vi "SamePrototype.vi"(4 "String To Append":string, 5 "Number To Multiply":dbl format="%.2f", 6 "Cluster In":T1 {"Numeric" format="%.2f"}, 7 "Array In":dbl[](array[numeric]) format="%.2f", 8 "String In":string, 9 "Numeric In":dbl format="%.2f") -> (0 "Cluster Out":T1 {"Numeric" format="%.2f"}, 1 "Array Out":dbl[](array[numeric]) format="%.2f", 2 "String Out":string, 3 "Numeric Out":dbl format="%.2f")   [LabVIEW 2012]
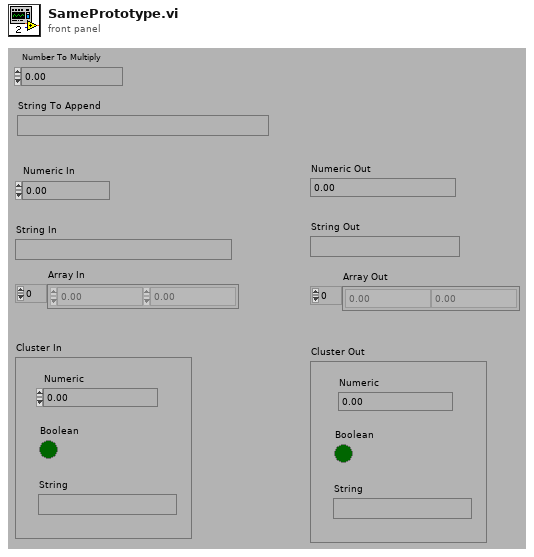
[diagram p1: front panel]
types:
  T1 = cluster{"Numeric":dbl, "Boolean":bool, "String":string}
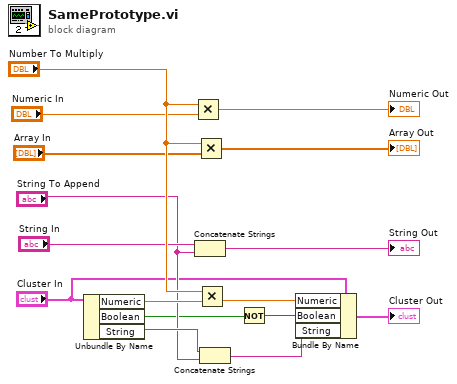
[diagram p0: block diagram]
diagram:
  n1 = Unbundle By Name("Cluster In") -> ("Numeric"=w15:dbl, "Boolean"=w7:bool, "String"=w9:string)
  n2 = Multiply(x="Number To Multiply", y="Numeric In") -> (x*y=→"Numeric Out":dbl)
  n3 = Concatenate Strings("String In", "String To Append") -> (→"String Out":string)
  n4 = Multiply(x="Number To Multiply", y="Array In") -> (x*y=→"Array Out":dbl[])
  n5 = Multiply(x="Number To Multiply", y=w15) -> (x*y=w4:dbl)
  n6 = Concatenate Strings(w9, "String To Append") -> (w3:string)
  n7 = Not(x=w7) -> (.not. x?=w5:bool)
  n8 = Bundle By Name(cluster="Cluster In", "Numeric"=w4, "Boolean"=w5, "String"=w3) -> (→"Cluster Out":T1)
